vi "Sub_Stiffen_Pin_Location.vi"(10 "Pre-Pin Matrix":dbl[][](array[numeric])) -> (3 "Post-Pin Matrix":dbl[][](array[numeric]))   [LabVIEW 2019]
uses:
  <vilib>/Analysis/Matrix/Numeric/Conversions/Matrix To Array - RM.vi
  <vilib>/Analysis/Matrix/NI_Matrix.lvlib
panel:
  in  "Pin Location":i32
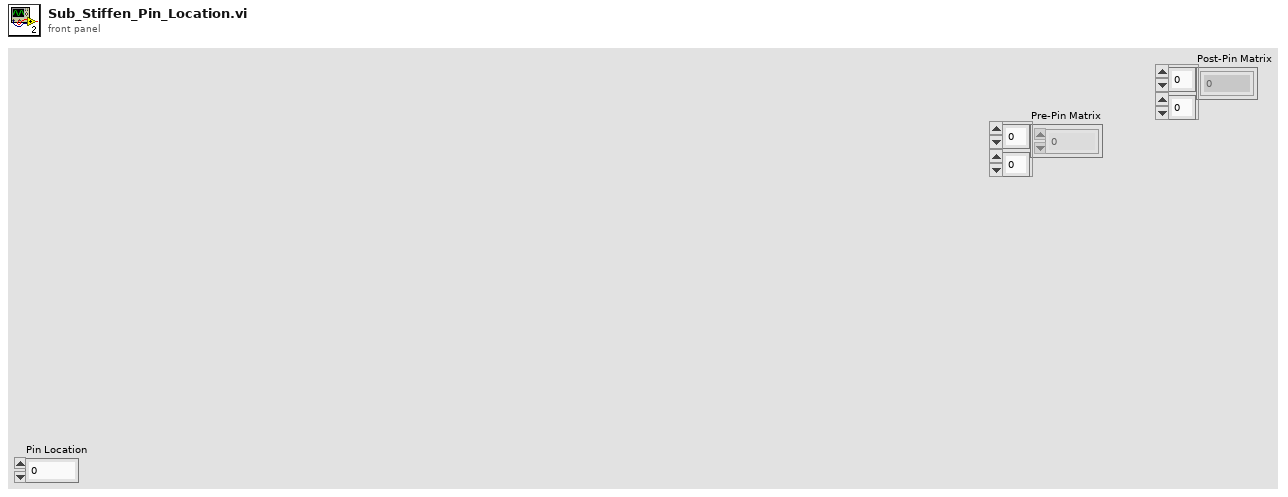
[diagram p1: front panel]
types:
  T1 = typedef "NI_Matrix.lvlib/RealMatrix.ctl" = dbl[][]
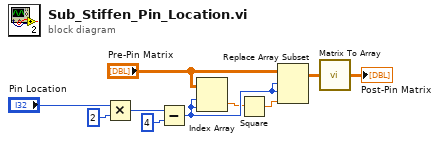
[diagram p0: block diagram]
diagram:
  n1 = Multiply(x="Pin Location", y=2) -> (x*y=w8:i32)
  n2 = Subtract(x=w8, y=4) -> (x-y=w3:i32)
  n3 = Index Array(array="Pre-Pin Matrix", index (row)=w3, index (col)=w3) -> (element=w2:dbl)
  n4 = Square(x=w2) -> (x^2=w1:dbl)
  n5 = Replace Array Subset(array="Pre-Pin Matrix", new element=w1, index (row)=w3, index (col)=w3) -> (w6:T1)
  n6 = call-poly <vilib>:"Matrix To Array.vi"("Real Matrix"=w6) -> ("Real 2D Array"=→"Post-Pin Matrix":dbl[][])
